vi "Diagnostic Logger v1.6.vi"() -> ()   [LabVIEW 2014]
uses:
  <vilib>/Rock Robotics/WPI/DriverStation/WPI_DriverStationRobotMode2.ctl
  <vilib>/Utility/file.llb/Write To Spreadsheet File (DBL).vi
  Begin/Global Variables.vi
panel:
  out "nRef":refnum<notifier>
  # "CSV Columns Transposed:\n\n01 - Robot Mode (0=?, 1=Auton, 2=Teleop)\n02 - Elapsed Time (ms)\n03 - dt (ms)\n04 - Gyro Yaw\n05 - Gyro Pitch\n06 - Gyro Roll\n07 - Driver JS LX\n08 - Driver JS LY\n09 - Driver JS RX\n10 - Drive Resolver FL\n11 - Drive Resolver FR\n12 - Drive Resolver BL\n13 - Drive Resolver BR\n14 - Drive Encoder FL\n15 - Drive Encoder FR\n16 - Drive Encoder BL\n17 - Drive Encoder BR\n18 - Drive Speed FL\n19 - Drive Speed FR\n20 - Drive Speed BL\n21 - Drive Speed BR\n22 - Lift Height Left\n23 - Lift Height Right\n24 - Lift Rate Left\n25 - Lift Rate Right"
  # "Data Usage Rates:\n\n20 KB / sec\n1.2 MB / min\n72 MB / hour"
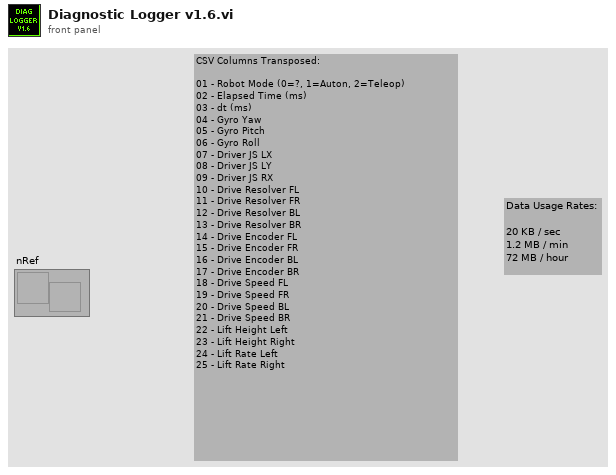
[diagram p1: front panel]
types:
  T1 = typedef "WPI_DriverStationRobotMode2.ctl" = enum16{"Autonomous Disabled", "Autonomous Enabled", "Teleop Disabled", "Teleop Enabled", "Disconnected", "Finish", "Test Disabled", "Test Enabled", "Emergency Stopped"}
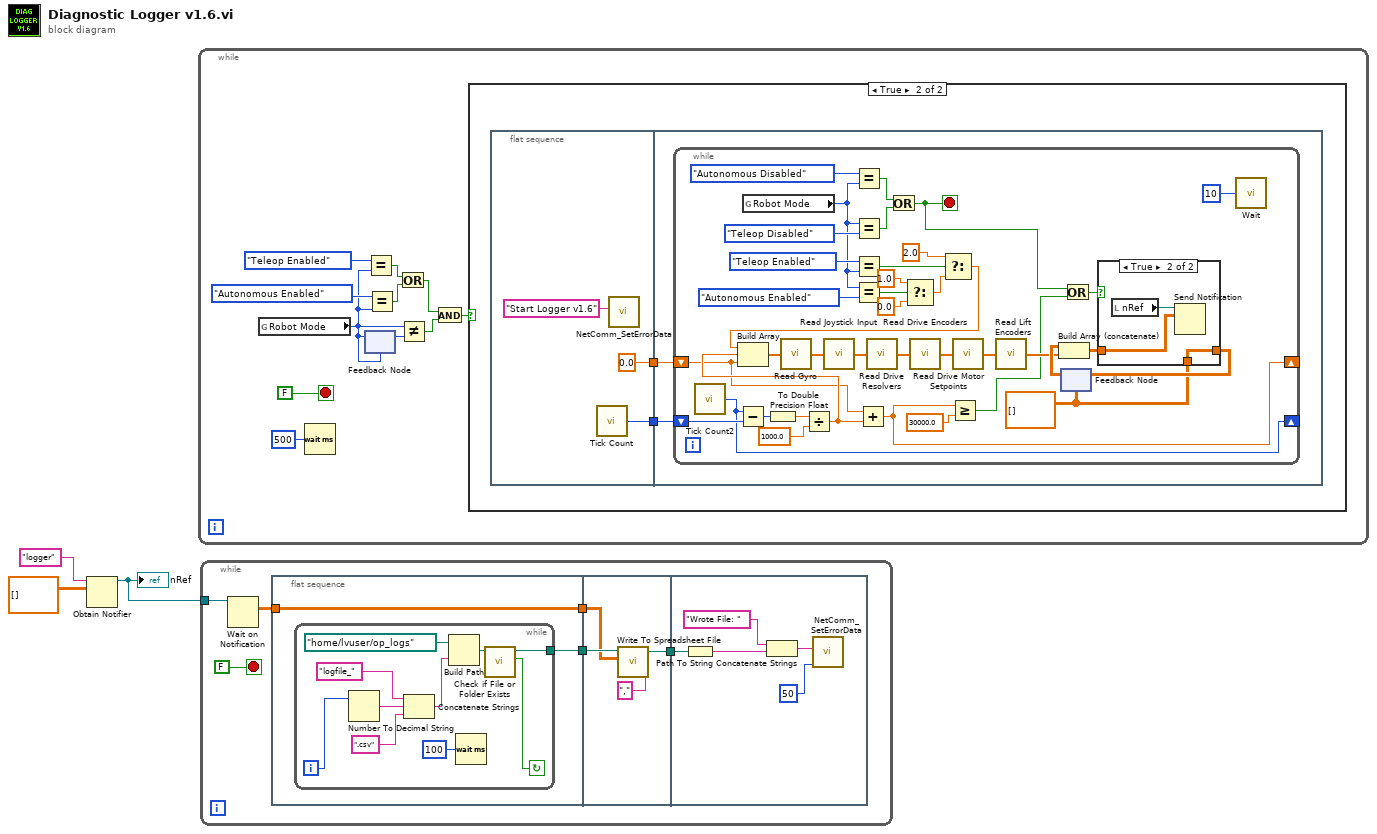
[diagram p0: block diagram]
diagram:
  n1 = Obtain Notifier(name (unnamed)="logger", notification data type=dbl[][] []) -> (notifier out=w1:refnum<notifier>)  [unwired: 2 in, 2 out]
  "nRef" <- w1
  n2 = while {
    stop <- FALSE stop-if-true
    n3 = global read "Global Variables.vi" "Robot Mode"() -> (w9:T1)
    n4 = Wait (ms)(milliseconds to wait=u32 500) -> ()  [unwired: 1 out]
    n5 = feedback-in #1(w9) -> ()
    n6 = feedback #1(w9) -> (w13:T1)
    n7 = Equal?(x=WPI_DriverStationRobotMode2."Teleop Enabled", y=w9) -> (x = y?=w8:bool)
    n8 = Equal?(x=WPI_DriverStationRobotMode2."Autonomous Enabled", y=w9) -> (x = y?=w7:bool)
    n9 = Or(x=w8, y=w7) -> (x .or. y?=w6:bool)
    n10 = Not Equal?(x=w9, y=w13) -> (x != y?=w12:bool)
    n11 = And(x=w6, y=w12) -> (x .and. y?=w5:bool)
    n12 = case shown="True" w5 {
      frame False {
      }
      frame True {
        n13 = flat-sequence {
          tunnel: [w18] -> w16
          tunnel: [0.0] -> w15
          tunnel: w16 -> [w21]
          tunnel: w15 -> [w20]
          frame #0 {
            n14 = call "Tick Count"() -> ("Tick Count(uSec)"=w18:u32)
            n15 = call <vilib>:"NetComm_SetErrorData.vi"("Error Data"="Start Logger v1.6") -> ()  [unwired: 3 in, 8 out]
          }
          frame #1 {
            n16 = while {
              shift-right: [w30] -> _
              shift-left: w21 -> [w31]
              shift-right: [w24] -> _
              shift-left: w20 -> [w25]
              stop <- w32 stop-if-true
              w35 = dbl[][] []
              n17 = call "Tick Count2"() -> ("Tick Count(uSec)"=w30:u32)
              n18 = Subtract(x=w30, y=w31) -> (x-y=w29:u32)
              n19 = global read "Global Variables.vi" "Robot Mode"() -> (w52:T1)
              n20 = To Double Precision Float(number=w29) -> (double precision float=w28:dbl)
              n21 = Divide(x=w28, y=1000.0) -> (x/y=w26:dbl)
              n22 = Equal?(x=WPI_DriverStationRobotMode2."Autonomous Disabled", y=w52) -> (x = y?=w56:bool)
              n23 = Equal?(x=w52, y=WPI_DriverStationRobotMode2."Teleop Disabled" ("x")) -> (x = y?=w57:bool)
              n24 = Equal?(x=WPI_DriverStationRobotMode2."Teleop Enabled", y=w52) -> (x = y?=w54:bool)
              n25 = Equal?(x=w52, y=WPI_DriverStationRobotMode2."Autonomous Enabled" ("x")) -> (x = y?=w51:bool)
              n26 = Add(x=w25, y=w26) -> (x+y=w24:dbl)
              n27 = Or(x=w56, y=w57) -> (x .or. y?=w32:bool)
              n28 = Select(t=1.0, s=w51, f=0.0) -> (s? t:f=w50:dbl)
              n29 = Select(t=2.0, s=w54, f=w50) -> (s? t:f=w39:dbl)
              n30 = Build Array(w39, w26, w25) -> (w40:dbl[])
              n31 = call "Read Gyro.vi"("Input Array"=w40) -> ("Appended Array"=w45:dbl[])
              n32 = call "Read Joystick Input.vi"("Input Array"=w45) -> ("Appended Array"=w44:dbl[])
              n33 = call "Read Drive Resolvers.vi"("Input Array"=w44) -> ("Appended Array"=w43:dbl[])
              n34 = call "Read Drive Encoders.vi"("Input Array"=w43) -> ("Appended Array"=w42:dbl[])  [unwired: 10 in, 4 out]
              n35 = Greater Or Equal?(x=w24, y=30000.0) -> (x >= y?=w22:bool)
              n36 = call "Read Drive Motor Setpoints.vi"("Input Array"=w42) -> ("Appended Array"=w41:dbl[])
              n37 = call "Read Lift Encoders.vi"("Input Array"=w41) -> ("Appended Array"=w38:dbl[])
              n38 = feedback #2(w35) -> (w46:dbl[][])
              n39 = Build Array (concatenate)(w46, w38) -> (w37:dbl[][])
              n40 = Or(x=w32, y=w22) -> (x .or. y?=w33:bool)
              n41 = case shown="True" w33 {
                tunnel: w37 -> [w60 w62]
                tunnel: [w60 w63] -> w36
                tunnel: w35 -> [_ w63]
                frame False {
                }
                frame True {
                  n42 = local read "nRef"() -> (w61:refnum<notifier>)
                  n43 = Send Notification(notification=w62, notifier=w61) -> ()  [unwired: 1 in, 2 out]
                }
              }
              n44 = feedback-in #2(w36) -> ()
              n45 = call "Wait"("Count(mSec)"=u32 10) -> ()  [unwired: 1 out]
            }
          }
        }
      }
    }
  }
  n46 = while {
    tunnel: w1 -> [w64]
    stop <- FALSE stop-if-true
    n47 = Wait on Notification(notifier=w64) -> (notification=w68:dbl[][])  [unwired: 3 in, 3 out]
    n48 = flat-sequence {
      tunnel: w68 -> [w71]
      tunnel: [w71] -> w67
      tunnel: [w70] -> w66
      tunnel: w67 -> [w83]
      tunnel: w66 -> [w84]
      tunnel: [w82] -> w65
      tunnel: w65 -> [w86]
      frame #0 {
        n49 = while {
          tunnel: [w74] -> w70
          i -> [w73]
          stop <- w81 continue-if-true
          n50 = Number To Decimal String(number=w73) -> (decimal integer string=w78:string)  [unwired: 1 in]
          n51 = Concatenate Strings("logfile_", w78, ".csv") -> (w77:string)
          n52 = Build Path(base path=path "/home/lvuser/op_logs" ("file path (dialog if empty)"), name or relative path=w77) -> (appended path=w80:path)
          n53 = Wait (ms)(milliseconds to wait=u32 100) -> ()  [unwired: 1 out]
          n54 = call <vilib>:"Check if File or Folder Exists.vi"("path"=w80) -> ("file or folder exists?"=w81:bool, "dup path"=w74:path)  [unwired: 8 in, 1 out]
        }
      }
      frame #1 {
        n55 = call-poly <vilib>:"Write To Spreadsheet File.vi"("delimiter (\\t)"="," ("delimiter (\\t)"), "2D data"=w83, "file path (dialog if empty)"=w84) -> ("new file path (Not A Path if cancelled)"=w82:path)  [unwired: 5 in]
      }
      frame #2 {
        n56 = Path To String(path=w86) -> (string=w87:string)
        n57 = Concatenate Strings("Wrote File: ", w87) -> (w89:string)
        n58 = call <vilib>:"NetComm_SetErrorData.vi"("Timeout (ms)"=50, "Error Data"=w89) -> ()  [unwired: 2 in, 8 out]
      }
    }
  }
